vi "sub3.vi"(11 "Terminal in":refnum<vi>) -> (3 "Argument":T1)   [LabVIEW 2020, in "CSM-Helper.lvclass"]
uses:
  CSM-Helper.lvclass
  Typedef/Def-Argument Info.ctl
  <userlib>/_OpenG.lib/string/string.llb/Trim Whitespace (String Array)__ogtk.vi
  <userlib>/_OpenG.lib/array/array.llb/Filter 1D Array (String)__ogtk.vi
  <userlib>/_OpenG.lib/array/array.llb/Filter 1D Array with Scalar (String)__ogtk.vi
  CSM-Helper.lvclass/CSM-Helper.ctl
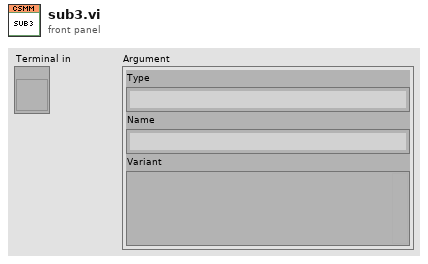
[diagram p1: front panel]
types:
  T1 = typedef "CSM-Helper.lvclass/Def-Argument Info.ctl" = cluster{"Type":string, "Name":string, "Variant":variant}
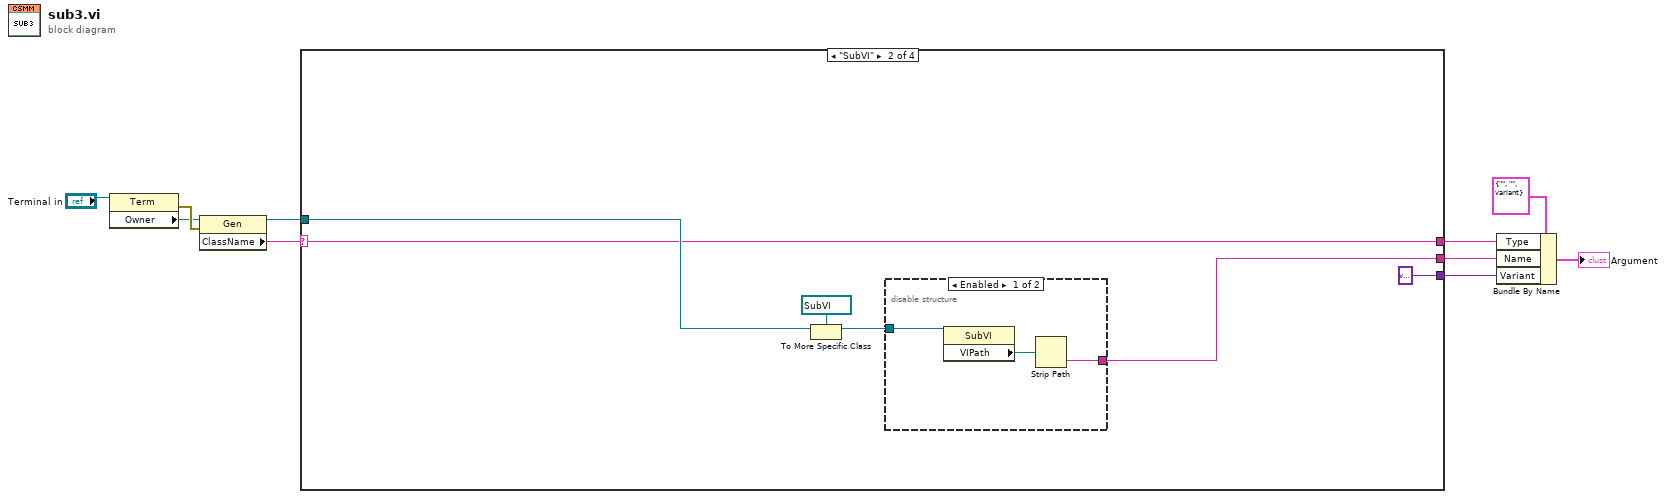
[diagram p0: block diagram]
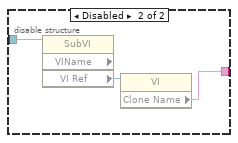
[diagram p3: hidden frame]
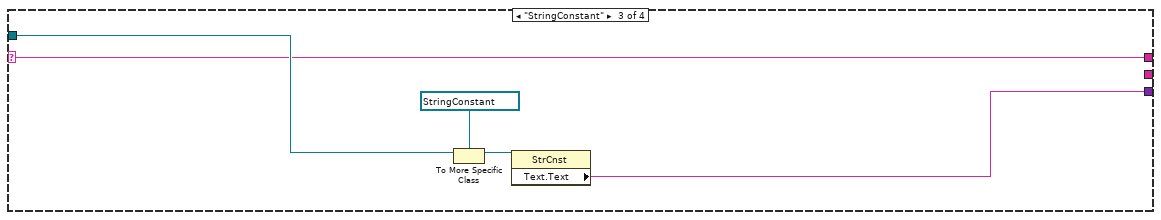
[diagram p4: hidden frame]
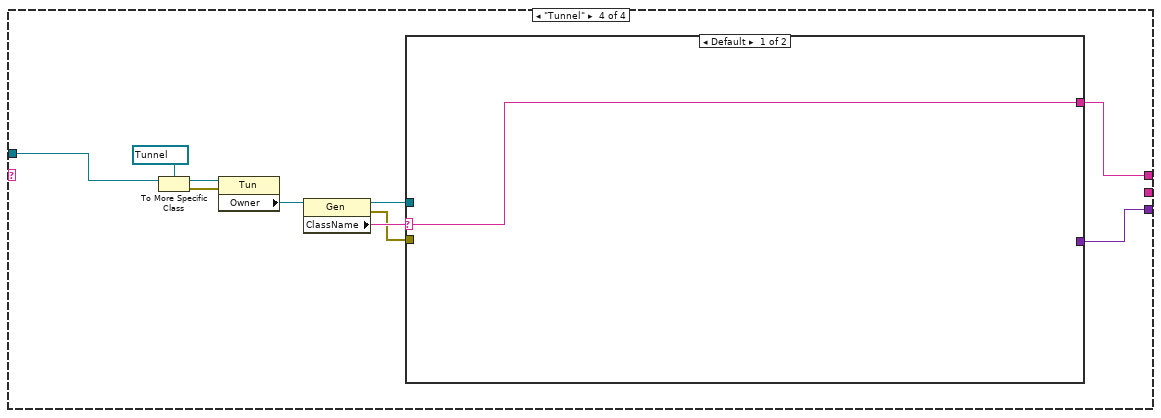
[diagram p5: hidden frame]
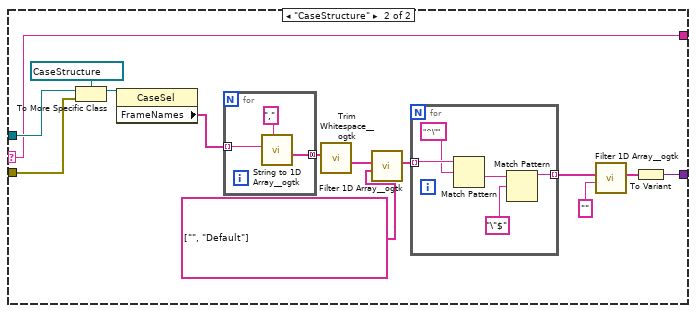
[diagram p6: hidden frame]
diagram:
  n1 = property class="Term"(reference="Terminal in") -> (error out=w5:errorcluster, "Owner"=w3:refnum<vi>)  [unwired: 1 in, 1 out]
  n2 = property class="Gen"(reference=w3, error in=w5) -> (reference out=w4:refnum<vi>, "ClassName"=w7:string)  [unwired: 1 out]
  n3 = case shown="\"SubVI\"" w7 {
    selector: w7 -> [w11 w12 w24 _]
    tunnel: w4 -> [_ w15 w26 w37]
    tunnel: [_ w14 _ _] -> w8
    tunnel: [_ variant w25 w38] -> w9
    tunnel: [w11 w12 w24 w29] -> w1
    frame Default {
    }
    frame "SubVI" {
      n4 = To More Specific Class(target class=refnum<vi> refnum ("reference out"), reference=w15) -> (specific class reference=w16:refnum<vi>)  [unwired: 1 in, 1 out]
      n5 = disable-structure "Diagram Disable Structure" shown="Enabled" {
        disable-tunnel: w16 -> [w20 w23]
        disable-tunnel: [w18 w21] -> w14
        frame Enabled {
          n6 = property class="SubVI"(reference=w20) -> ("VIPath"=w19:path)  [unwired: 1 in, 2 out]
          n7 = Strip Path(path=w19) -> (name=w18:string)  [unwired: 1 out]
        }
        frame Disabled {
          n8 = property class="SubVI" props=["VIName", "VI Ref"](reference=w23) -> ("VI Ref"=w22:refnum<vi>)  [unwired: 1 in, 3 out]
          n9 = property class="VI"(reference=w22) -> ("Clone Name"=w21:string)  [unwired: 1 in, 2 out]
        }
      }
    }
    frame "StringConstant" {
      n10 = To More Specific Class(target class=refnum<vi> refnum ("reference out"), reference=w26) -> (specific class reference=w28:refnum<vi>)  [unwired: 1 in, 1 out]
      n11 = property class="StrCnst"(reference=w28) -> ("Text.Text"=w25:string)  [unwired: 1 in, 2 out]
    }
    frame "Tunnel" {
      n12 = To More Specific Class(target class=refnum<vi> refnum ("reference out"), reference=w37) -> (specific class reference=w35:refnum<vi>, error out=w34:errorcluster)  [unwired: 1 in]
      n13 = property class="Tun"(reference=w35, error in=w34) -> ("Owner"=w33:refnum<vi>)  [unwired: 2 out]
      n14 = property class="Gen"(reference=w33) -> (reference out=w31:refnum<vi>, error out=w30:errorcluster, "ClassName"=w32:string)  [unwired: 1 in]
      n15 = case shown="Default" w32 {
        selector: w32 -> [w39 w40]
        tunnel: [_ w43] -> w38
        tunnel: w31 -> [_ w42]
        tunnel: w30 -> [_ w41]
        tunnel: [w39 w40] -> w29
        frame Default {
        }
        frame "CaseStructure" {
          n16 = To More Specific Class(target class=refnum<vi> refnum ("reference out"), reference=w42, error in=w41) -> (specific class reference=w53:refnum<vi>)  [unwired: 1 out]
          n17 = property class="CaseSel"(reference=w53) -> ("FrameNames"=w45:string[])  [unwired: 1 in, 2 out]
          n18 = for {
            tunnel: [w60] -> w48 mode=concatenating
            tunnel: w45 -> [w59] mode=indexing
            n19 = call <userlib>:"String to 1D Array__ogtk.vi"("delimiter (Tab)"=",", "string"=w59) -> ("Array of Strings"=w60:string[])  [unwired: 9 in]
          }
          n20 = call-poly <userlib>:"Trim Whitespace__ogtk.vi"("String in"=w48) -> ("String out"=w49:string[])  [unwired: 6 in]
          n21 = call-poly <userlib>:"Filter 1D Array__ogtk.vi"("items to filter"=string[] ["", "Default"], "array"=w49) -> ("filtered array"=w50:string[])  [unwired: 4 in, 1 out]
          n22 = for {
            tunnel: w50 -> [w58] mode=indexing
            tunnel: [w54] -> w51 mode=indexing
            n23 = Match Pattern(string=w58, regular expression="^\"") -> (after substring=w56:string)  [unwired: 1 in, 3 out]
            n24 = Match Pattern(string=w56, regular expression="\"$") -> (before substring=w54:string)  [unwired: 1 in, 3 out]
          }
          n25 = call-poly <userlib>:"Filter 1D Array__ogtk.vi"("items to filter"="" ("String"), "array"=w51) -> ("filtered array"=w44:string[])  [unwired: 4 in, 1 out]
          n26 = To Variant(anything=w44) -> (Variant=w43:variant)
        }
      }
    }
  }
  n27 = Bundle By Name(cluster=T1 {"Type"="", "Name"="", "Variant"=variant} ("Argument"), "Type"=w1, "Name"=w8, "Variant"=w9) -> (→"Argument":T1)
